vi "G4BaseTemplate_Singleton_4x4x4_WriteAttribute.vi"(8 "Error In":errorcluster) -> (0 "Error Out":errorcluster)   [LabVIEW 2020]
uses:
  <resource>/Framework/Providers/Open_GDS/ClassProviders/Provider_EndevoGOOP400/Templates/G4BaseTemplate_Singleton_4x4x4/G4BaseTemplate_Singleton_4x4x4.lvclass
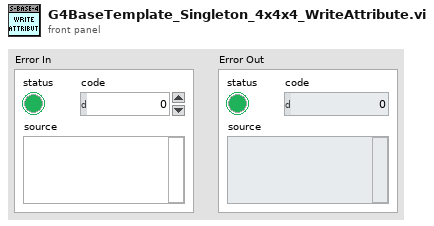
[diagram p1: front panel]
types:
  T1 = typedef "G4BaseTemplate_Singleton_4x4x4.lvclass/ObjectAttributes.ctl" = cluster{"Attribute1":dbl}
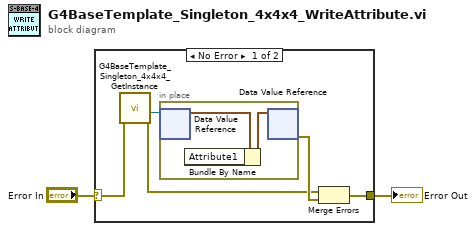
[diagram p0: block diagram]
diagram:
  n1 = case shown="No Error" "Error In" {
    selector: "Error In" -> [w7 w10]
    tunnel: [w3 w10] -> w1
    frame No Error {
      n2 = call <resource>:"G4BaseTemplate_Singleton_4x4x4_GetInstance.vi"("error in (no error)"=w7) -> ("error out"=w4:errorcluster, "DVRRefOut"=w5:refnum<data-value>)  [unwired: 6 in, 3 out]
      n3 = in-place {
        n4 = in-place-dvr #1(w5) -> (w8:T1)  [unwired: 1 out]
        n5 = Bundle By Name(cluster=w8) -> (w9:T1)  [unwired: 1 in]
        n6 = in-place-dvr #1(w9) -> (w6:errorcluster)  [unwired: 1 out]
      }
      n7 = Merge Errors(w4, w6) -> (w3:errorcluster)
    }
    frame Error {
    }
  }
  "Error Out" <- w1
